vi "Common_Py_Compare_Image.vi"(0 "session in":refnum<k35>, 5 "module path":path=path "D:/dev/Guy_Storage/Work/Cancun/MW_Display_Test/Magewell Capture/Capture_LV.py", 11 "error in":errorcluster, 12 "Input":T1) -> (4 "session out":refnum<k35>, 6 "module path out":path, 14 "Done":bool, 15 "error out":errorcluster)   [LabVIEW 2023]
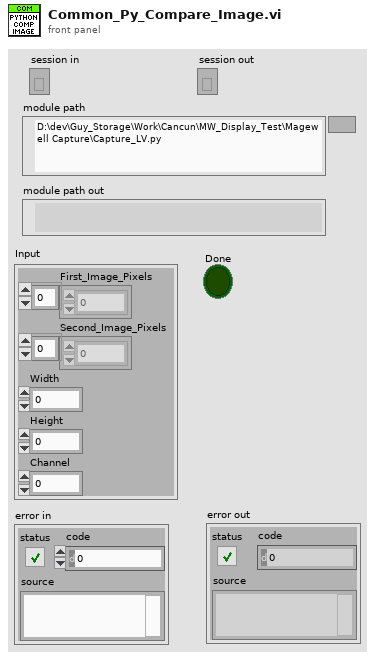
[diagram p1: front panel]
types:
  T1 = cluster{"First_Image_Pixels":u8[], "Second_Image_Pixels":u8[], "Width":i32, "Height":i32, "Channel":i32}
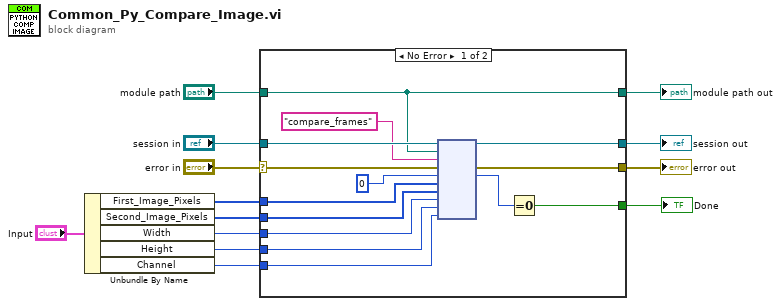
[diagram p0: block diagram]
diagram:
  n1 = Unbundle By Name("Input") -> ("First_Image_Pixels"=w5:u8[], "Second_Image_Pixels"=w4:u8[], "Width"=w3:i32, "Height"=w2:i32, "Channel"=w1:i32)
  n2 = case shown="No Error" "error in" {
    selector: "error in" -> [w24 w29]
    tunnel: "module path" -> [w22 w28]
    tunnel: "session in" -> [w27 w30]
    tunnel: [w26 w29] -> w9
    tunnel: [w25 w30] -> w11
    tunnel: [w22 w28] -> w8
    tunnel: [w19 _] -> w7
    tunnel: w5 -> [w18 _]
    tunnel: w4 -> [w17 _]
    tunnel: w3 -> [w16 _]
    tunnel: w2 -> [w15 _]
    tunnel: w1 -> [w14 _]
    frame No Error {
      n3 = node(w27, w22, "compare_frames" ("function name"), w24, 0, w18, w17, w16, w15, w14) -> (w25:refnum<k35>, w26:errorcluster, w20:i32)  [unwired: 5 in, 2 out]
      n4 = Equal To 0?(x=w20) -> (x = 0?=w19:bool)
    }
    frame Error {
    }
  }
  "session out" <- w11
  "error out" <- w9
  "module path out" <- w8
  "Done" <- w7
